vi "四舍五入取整.vi"(11 "x":i8) -> (3 "x*y":i8)   [LabVIEW 2016, in "斯坦道CODMn.lvlib"]
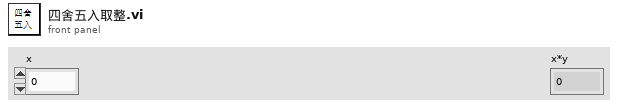
[diagram p1: front panel]
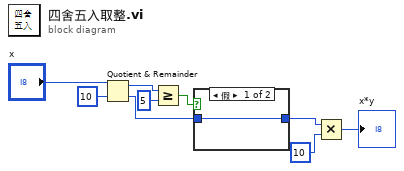
[diagram p0: block diagram]
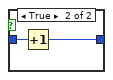
[diagram p2: hidden frame]
diagram:
  n1 = Quotient & Remainder(x="x", y=i8 10) -> (x-y*floor(x/y)=w3:i8, floor(x/y)=w1:i8)
  n2 = Greater Or Equal?(x=w3, y=i8 5) -> (x >= y?=w2:bool)
  n3 = case shown="假" w2 {
    tunnel: w1 -> [w10 w12]
    tunnel: [w10 w11] -> w7
    frame False {
    }
    frame True {
      n4 = Increment(x=w12) -> (x+1=w11:i8)
    }
  }
  n5 = Multiply(x=w7, y=i8 10) -> (x*y=→"x*y":i8)
